vi "chart series set trendline line.vi"(8 "error in (no error)":errorcluster, 10 "line":T1, 11 "series":u32) -> (0 "error out":errorcluster, 2 "line out":T1, 3 "function return":u32(ring))   [LabVIEW 2015, in "xlsxwriter.lvlib"]
doc: "lxw_error chart_series_set_trendline_line(lxw_chart_series series, lxw_chart_line *line);"
uses:
  xlsxwriter.lvlib
  xlsxwriter.dll
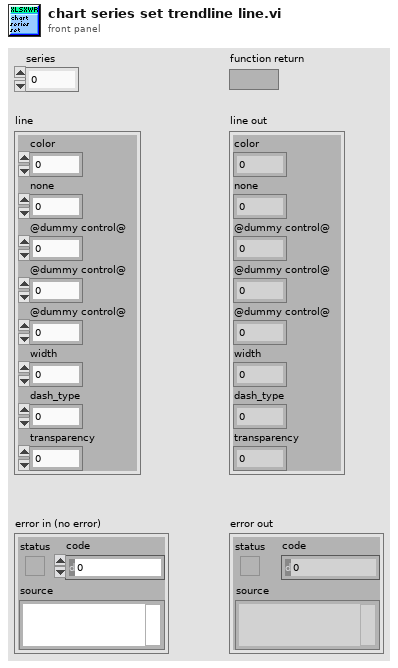
[diagram p1: front panel]
types:
  T1 = cluster{"color":u32, "none":u8, "@dummy control@":i8, "@dummy control@":i8, "@dummy control@":i8, "width":sgl, "dash_type":u8, "transparency":u8}
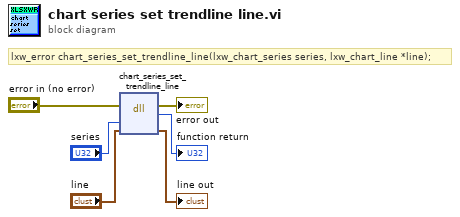
[diagram p0: block diagram]
diagram:
  # "lxw_error chart_series_set_trendline_line(lxw_chart_series series, lxw_chart_line *line);"
  n1 = dll-call lib="C:/Users/WDAGUtilityAccount/Desktop/lv_vis_added_cell/xlsxwriter.*" fn="chart_series_set_trendline_line"(error in="error in (no error)", "series"="series", "line"="line") -> (error out=→"error out":errorcluster, →"function return":u32, "line"=→"line out":T1)  [unwired: 3 in, 1 out]
